vi "Global_Cal Info.vi"() -> ()   [LabVIEW 2020]
uses:
  Support/Controls/Clst_Cal Info Global.ctl
  Support/Controls/Clst_Atm Info Global.ctl
panel:
  out "SubPnl Load Check wait?":bool
  out "SPEC error?":bool[](array[boolean])
  out "분해능적용?":bool=TRUE
  out "Func error?":bool[](array[boolean])
  in  "기타정보":cluster{"부서코드":string, "제조사코드":string}
  in  "User Input_str":string
  in  "불확도 유효자리":string="0"
  out "Spec변경?":bool[](array[boolean])
  out "std error?":bool[][](array[boolean])
  out "Func Use?":bool[](array[boolean])
  out "불러오기?":bool
  in  "Func List":string[][](array[string])
  in  "룸구분":string[][](table)=[["0", "A", "301", "302", "401", "402", "403", "404", "N03", "N04", "000"], ["0", "B", "101", "102", "103", "104", "105", "106", "N01", "", ""], ["0", "C", "701", "N07", "", "", "", "", "", "", ""], ["0", "D", "501", "502", "503", "N05", "", "", "", "", ""], ["0", "F", "", "", "", "", "", "", "", "", ""], ["0", "G", "901", "N09", "", "", "", "", "", "", ""], ["0", "H", "601", "603", "N06", "", "", "", "", "", ""], ["0", "K", "201", "40215", "N02", "", "", "", "", "", ""], ["0", "N", "", "", "", "", "", "", "", "", ""], ["0", "O", "406", "", "", "", "", "", "", "", ""], ["0", "P", "407", "", "", "", "", "", "", "", ""], ["0", "Q", "40703", "", "", "", "", "", "", "", ""], ["0", "R", "", "", "", "", "", "", "", "", ""], ["0", "S", "209", "", "", "", "", "", "", "", ""], ["0", "T", "202", "203", "204", "", "", "", "", "", ""], ["0", "U", "405", "", "", "", "", "", "", "", ""], ["0", "V", "", "", "", "", "", "", "", "", ""], ["5", "A", "10615", "10622", "", "", "", "", "", "", ""], ["4", "A", "", "", "", "", "", "", "", "", ""]]
  in  "교정환경":T1
  in  "교정절차":T2
  in  "교정자정보":cluster{"사번":string, "이름":string, "자격":string}
  out "교정정보":T3
  # "func"
  # "funcnam"
  # "func_ext"
  # "func_extnam"
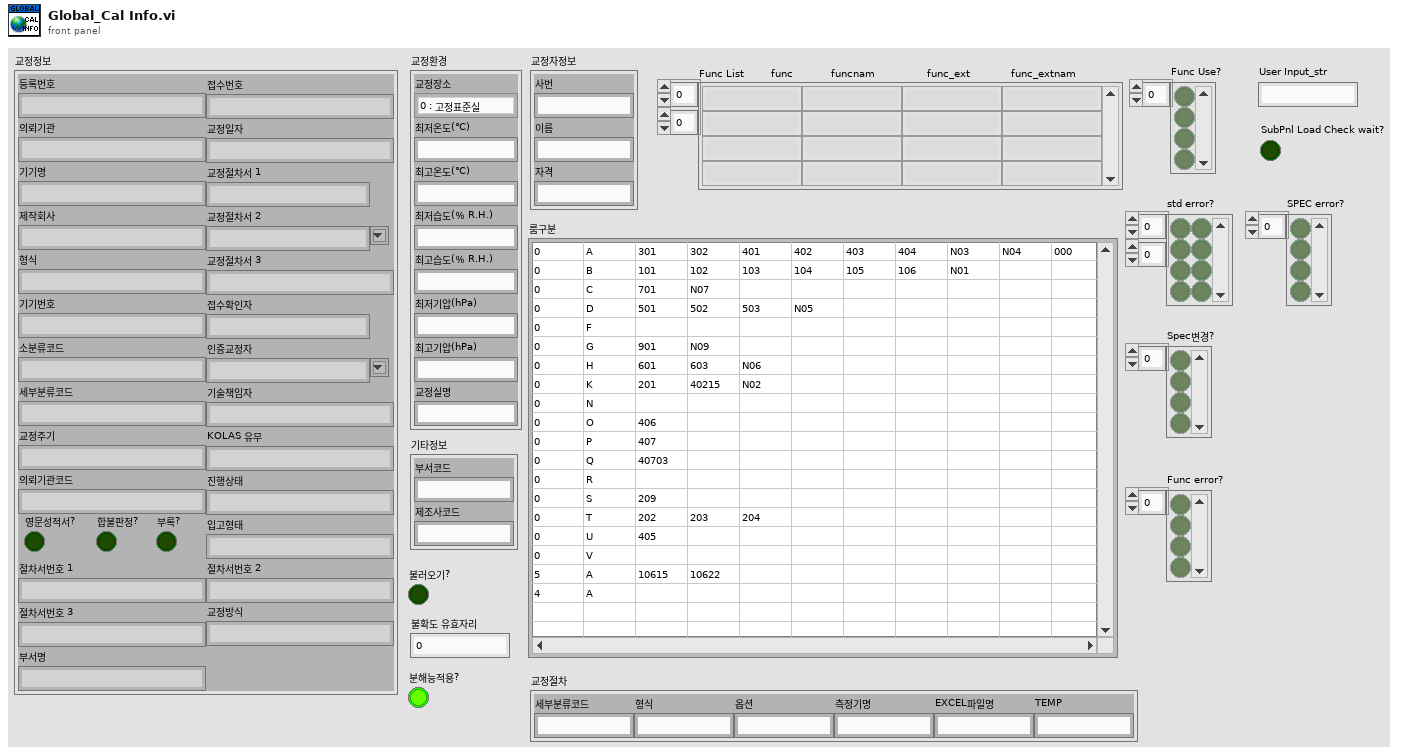
[diagram p1: front panel]
types:
  T1 = typedef "Clst_Atm Info Global.ctl" = cluster{"교정장소":enum16{"0 : 고정표준실", "1 : 현장교정"}, "최저온도(℃)":string, "최고온도(℃)":string, "최저습도(％ R.H.)":string, "최고습도(％ R.H.)":string, "최저기압(hPa)":string, "최고기압(hPa)":string, "교정실명":string}
  T2 = cluster{"세부분류코드":string, "형식":string, "옵션":string, "측정기명":string, "EXCEL파일명":string, "TEMP":string}
  T3 = typedef "Clst_Cal Info Global.ctl" = cluster{"등록번호":string, "의뢰기관":string, "기기명":string, "제작회사":string, "형식":string, "기기번호":string, "소분류코드":string, "세부분류코드":string, "교정주기":string, "접수번호":string, "교정일자":string, "교정절차서 1":string, "교정절차서 2":string, "교정절차서 3":string, "접수확인자":string, "인증교정자":string, "기술책임자":string, "KOLAS 유무":string, "진행상태":string, "의뢰기관코드":string, "입고형태":string, "영문성적서?":bool, "합불판정?":bool, "부록?":bool, "절차서번호 1":string, "절차서번호 2":string, "절차서번호 3":string, "교정방식":string, "부서명":string}
diagram:
